vi "Stop Acquisition.vi"(8 "error in (no error)":errorcluster, 11 "HW Refnum":string) -> (0 "error out":errorcluster)   [LabVIEW 2018, in "LGP5 Acquisition.lvlib" / "DAQ Device.lvlib"]
doc: "Stops the acquisition.\n_____\nBased on Delacor QMH Project Template 4.2.0.62."
uses:
  DAQ Device.lvlib
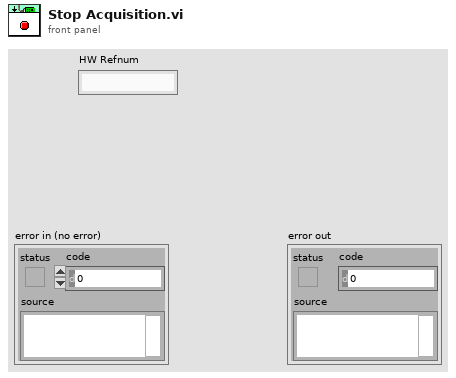
[diagram p1: front panel]
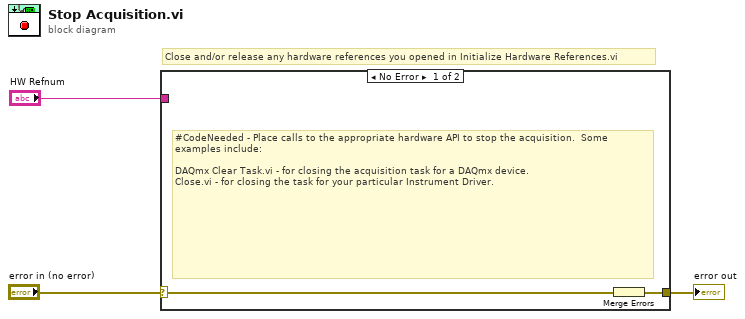
[diagram p0: block diagram]
diagram:
  # "Close and/or release any hardware references you opened in Initialize Hardware References.vi"
  n1 = case shown="No Error" "error in (no error)" {
    selector: "error in (no error)" -> [w4 w6]
    tunnel: [w5 w6] -> w2
    tunnel: "HW Refnum" -> [_ _]
    frame No Error {
      # "#CodeNeeded - Place calls to the appropriate hardware API to stop the acquisition.  Some examples include:\n\nDAQmx Clear Task.vi - for closing the acquisition task for a DAQmx device.\nClose.vi - for closing the task for your particular Instrument Driver."
      n2 = Merge Errors(w4) -> (w5:errorcluster)
    }
    frame Error {
    }
  }
  "error out" <- w2
